vi "Get Control Values.vi"(8 "error in (no error)":errorcluster, 11 "Hardware Game Pad Interface in":refnum<class "Hardware Game Pad Interface.lvclass">) -> (0 "error out":errorcluster, 2 "Cluster":T3, 3 "Hardware Game Pad Interface out":refnum<class "Hardware Game Pad Interface.lvclass">)   [LabVIEW 2017, in "Hardware Game Pad Interface.lvclass"]
uses:
  Hardware Game Pad Interface.lvclass
  Abstract Game Pad Interface/Game Pad Descriptor.ctl
  Hardware Game Pad Interface.lvclass/Hardware Game Pad Interface.ctl
  <vilib>/Utility/inputDevices.llb/joystickAcquire.vi
  Abstract Game Pad Interface/Abstract Game Pad Interface.lvclass
panel:
  out "axis info":T1
  out "button info":T2
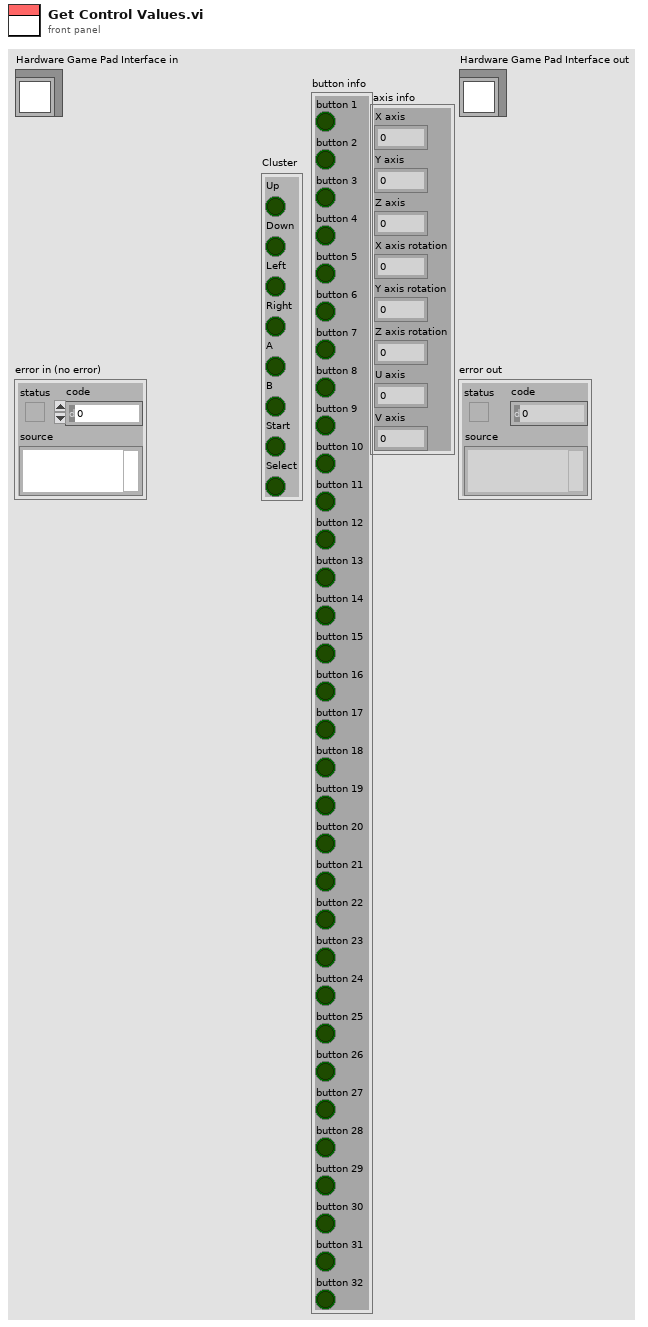
[diagram p1: front panel]
types:
  T1 = cluster{"X axis":i32, "Y axis":i32, "Z axis":i32, "X axis rotation":i32, "Y axis rotation":i32, "Z axis rotation":i32, "U axis":i32, "V axis":i32}
  T2 = cluster{"button 1":bool, "button 2":bool, "button 3":bool, "button 4":bool, "button 5":bool, "button 6":bool, "button 7":bool, "button 8":bool, "button 9":bool, "button 10":bool, "button 11":bool, "button 12":bool, "button 13":bool, "button 14":bool, "button 15":bool, "button 16":bool, "button 17":bool, "button 18":bool, "button 19":bool, "button 20":bool, "button 21":bool, "button 22":bool, "button 23":bool, "button 24":bool, "button 25":bool, "button 26":bool, "button 27":bool, "button 28":bool, "button 29":bool, "button 30":bool, "button 31":bool, "button 32":bool}
  T3 = typedef "Abstract Game Pad Interface.lvclass/Game Pad Descriptor.ctl" = cluster{"Up":bool, "Down":bool, "Left":bool, "Right":bool, "A":bool, "B":bool, "Start":bool, "Select":bool}
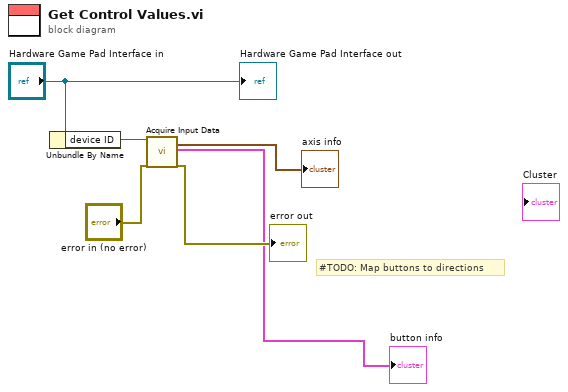
[diagram p0: block diagram]
diagram:
  # "#TODO: Map buttons to directions"
  n1 = Unbundle By Name("Hardware Game Pad Interface in") -> ("device ID"=w5:refnum<k1>)
  n2 = call-poly <vilib>:"Acquire Input Data.vi"("device ID"=w5, "error in (no error)"="error in (no error)") -> ("axis info"=→"axis info":T1, "button info"=→"button info":T2, "error out"=→"error out":errorcluster)  [unwired: 13 in, 2 out]
  "Hardware Game Pad Interface out" <- "Hardware Game Pad Interface in"
